vi "Evaluate.vi"(8 "error in (no error)":errorcluster, 10 "OSSP_Problem.lvclass":refnum<class "OSSP_Problem.lvclass">, 11 "GA in":refnum<class "GA.lvclass">) -> (0 "error out":errorcluster, 2 "OSSP_Problem out":refnum<class "OSSP_Problem.lvclass">, 3 "GA out":refnum<class "GA.lvclass">)   [LabVIEW 2013, in "GA.lvclass"]
uses:
  GA.lvclass
  OSSP_Problem.lvclass
  GA.lvclass/GA.ctl
  GA_Operation_To_MachineJobTuple.vi
  Find Gaps On Particular Machine.vi
  GA_Check_Other_Machines.vi
  GA_Schedule_Job.vi
  GA_Find_Job_On_Other_Machines.vi
  GA_Increment_NumberofJobsOn Machine_ByOne.vi
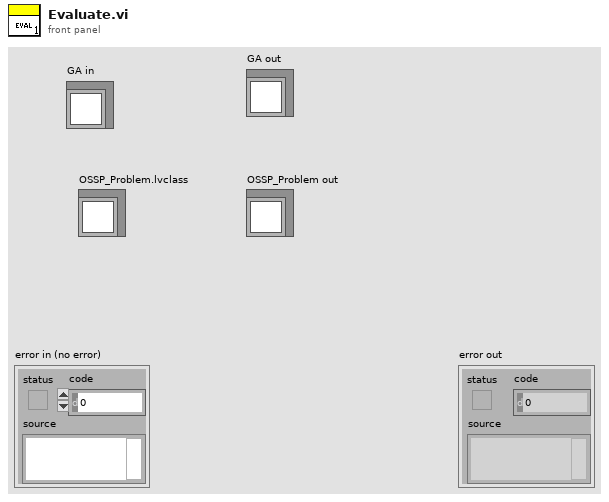
[diagram p1: front panel]
types:
  T1 = typedef "Solution.ctl" = cluster{"Schedule":u16[], "Fitness":u16, "Fitness Valid?":bool}
  T2 = typedef "GanntChart_Element.ctl" = cluster{"Operation Number":i32, "Job Number":i32, "Start Time":i32, "Procesing Time":u16, "End Time":i32}
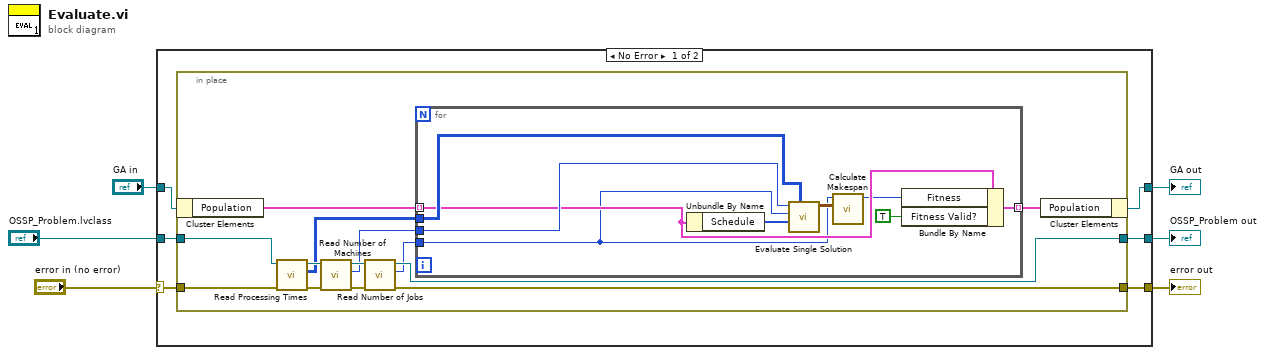
[diagram p0: block diagram]
diagram:
  n1 = case shown="No Error" "error in (no error)" {
    selector: "error in (no error)" -> [w11 w37]
    tunnel: [w10 w37] -> w5
    tunnel: [w7 w36] -> w3
    tunnel: "GA in" -> [w8 w36]
    tunnel: "OSSP_Problem.lvclass" -> [w12 w35]
    tunnel: [w9 w35] -> w1
    frame No Error {
      n2 = in-place {
        in-place-border: w12 -> [w25]
        in-place-border: w11 -> [w21]
        in-place-border: [w20] -> w10
        in-place-border: [w18] -> w9
        n3 = in-place-cluster #1(w8) -> ("Population"=w14:T1[])
        n4 = call-dynamic "Read Processing Times.vi"("error in (no error)"=w21, "OSSP_Problem in"=w25) -> ("error out"=w23:errorcluster, "Processing Times"=w17:u16[][], "OSSP_Problem out"=w24:refnum<class "OSSP_Problem.lvclass">)  [unwired: 7 in]
        n5 = call-dynamic "Read Number of Machines.vi"("error in (no error)"=w23, "OSSP_Problem in"=w24) -> ("error out"=w22:errorcluster, "Number of Machines"=w16:i32, "OSSP_Problem out"=w19:refnum<class "OSSP_Problem.lvclass">)  [unwired: 7 in]
        n6 = call-dynamic "Read Number of Jobs.vi"("error in (no error)"=w22, "OSSP_Problem in"=w19) -> ("error out"=w20:errorcluster, "Number of Jobs"=w15:i32, "OSSP_Problem out"=w18:refnum<class "OSSP_Problem.lvclass">)  [unwired: 7 in]
        n7 = for {
          tunnel: w14 -> [w31] mode=indexing
          tunnel: w16 -> [w33]
          tunnel: w15 -> [w26]
          tunnel: w17 -> [w34]
          tunnel: [w30] -> w13 mode=indexing
          n8 = Unbundle By Name(w31) -> ("Schedule"=w27:u16[])
          n9 = call "Evaluate Single Solution.vi"("Processing Times (Rows Mach.Cols Jobs)"=w34, "Schedule"=w27, "Number of Jobs"=w26, "Number of Machines"=w33) -> ("Gannt Chart Out"=w32:T2[][])  [unwired: 7 in]
          n10 = call "Calculate Makespan.vi"("Gannt Chart Out"=w32, "Number of Jobs"=w26) -> ("Makespan"=w29:i32)  [unwired: 9 in]
          n11 = Bundle By Name(cluster=w31, "Fitness"=w29, "Fitness Valid?"=TRUE) -> (w30:T1)
        }
        n12 = in-place-cluster #1("Population"=w13) -> (w7:refnum<class "GA.lvclass">)
      }
    }
    frame Error {
    }
  }
  "error out" <- w5
  "GA out" <- w3
  "OSSP_Problem out" <- w1
